vi "main.vi"() -> ()   [LabVIEW 2020]
uses:
  typedefs/typedef_stage_control.ctl
  typedefs/typedef_stage_position.ctl
panel:
  in  "stop":bool
  in  "Stage position":T1
  in  "Stage Control":T2={"Up"=FALSE, "Left"=FALSE, "Right"=FALSE, "Down"=FALSE, "Focus Down"=FALSE, "Focus Up"=FALSE, "X Step Size(um)"=100.0, "Z step size (um)"=100.0, "Y Step Size(um)"=100.0, "Enable x-axis"=TRUE, "Enable y-axis"=TRUE, "Enable z-axis"=TRUE, "Same step size"=FALSE, "Global step size"=0.0, "stop"=FALSE}
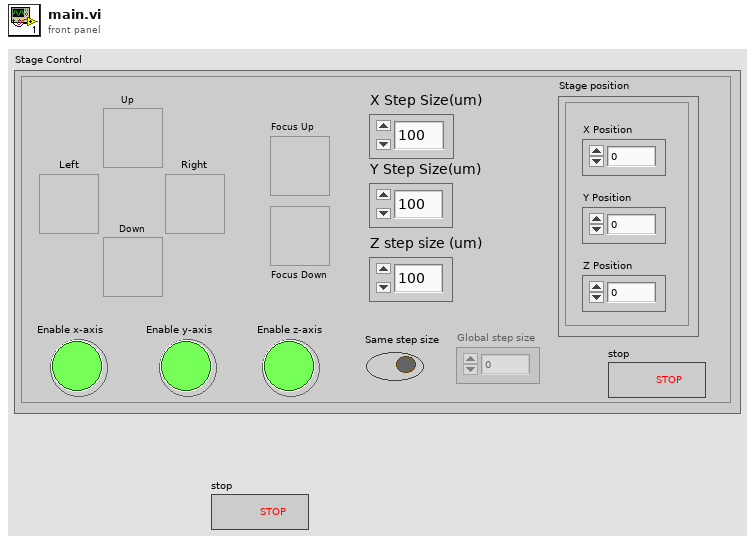
[diagram p1: front panel]
types:
  T1 = typedef "typedef_stage_position.ctl" = cluster{"X Position":dbl, "Y Position":dbl, "Z Position":dbl}
  T2 = typedef "typedef_stage_control.ctl" = cluster{"Up":bool, "Left":bool, "Right":bool, "Down":bool, "Focus Down":bool, "Focus Up":bool, "X Step Size(um)":dbl, "Z step size (um)":dbl, "Y Step Size(um)":dbl, "Enable x-axis":bool, "Enable y-axis":bool, "Enable z-axis":bool, "Same step size":bool, "Global step size":dbl, "stop":bool}
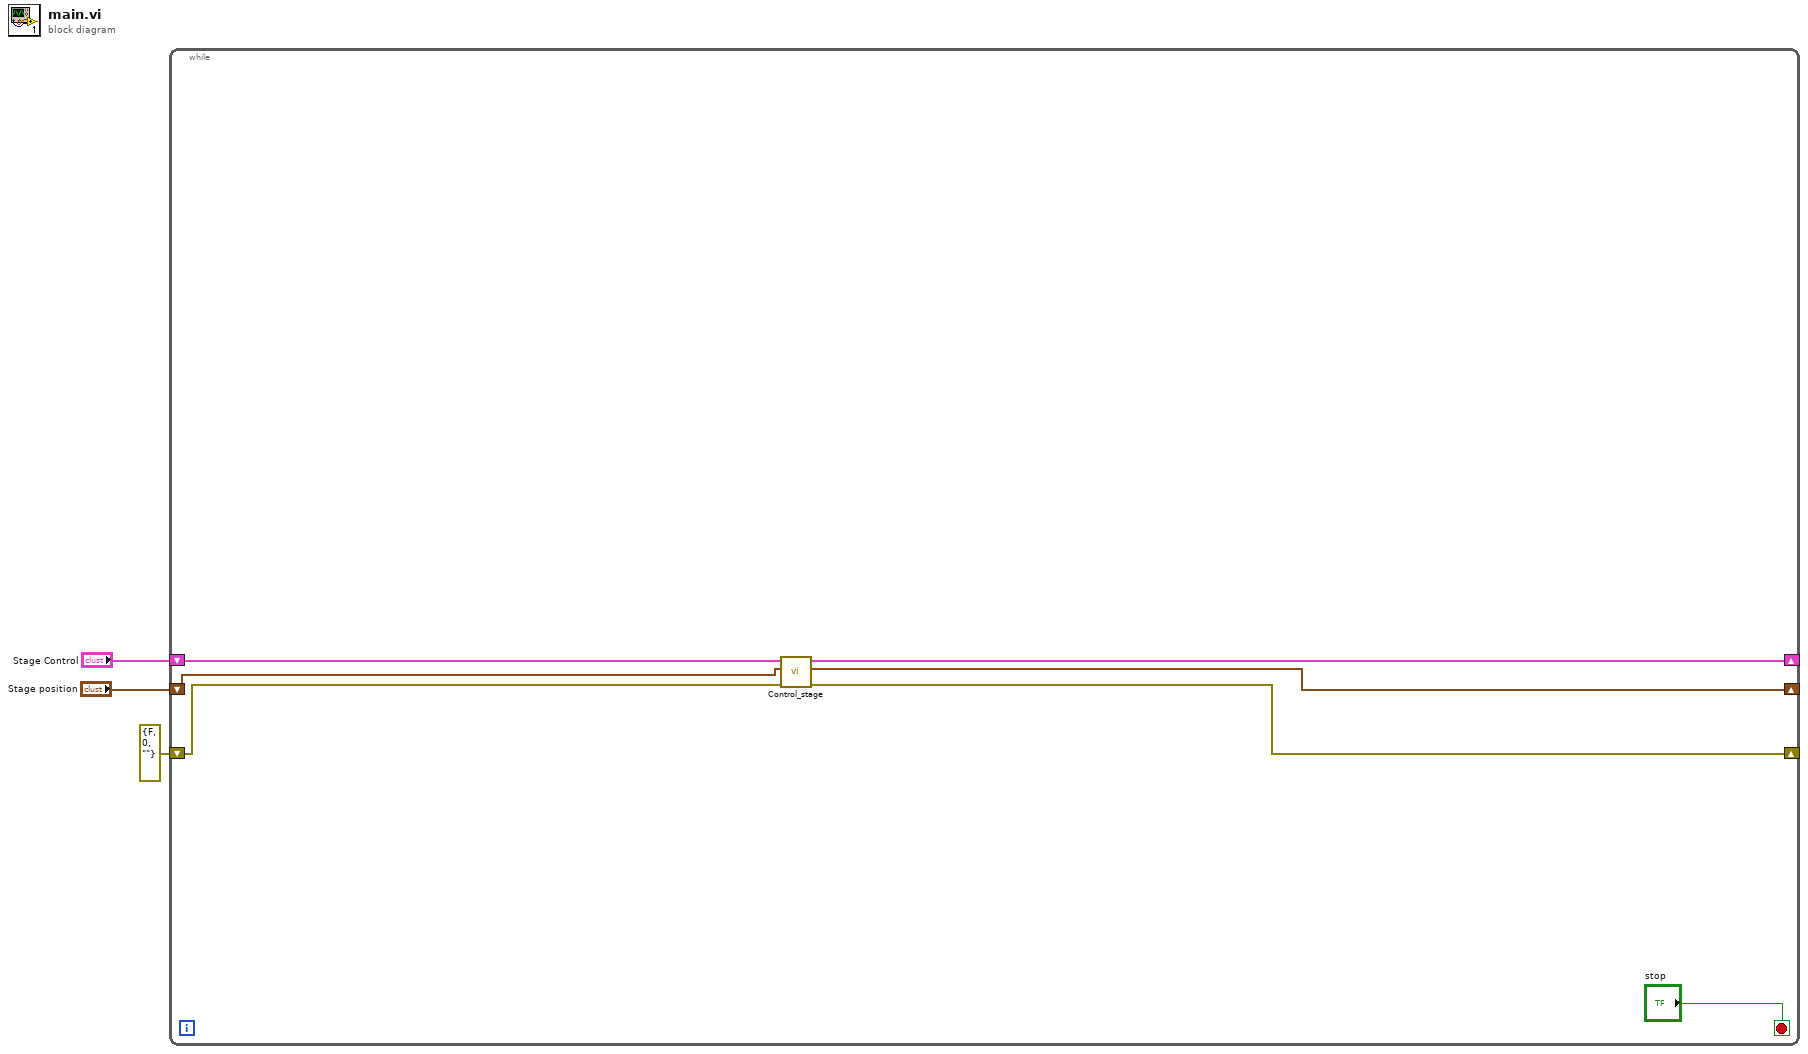
[diagram p0: block diagram]
diagram:
  n1 = while {
    shift-right: [w8] -> _
    shift-left: "Stage Control" -> [w10]
    shift-right: [w7] -> _
    shift-left: "Stage position" -> [w9]
    shift-right: [w6] -> _
    shift-left: errorcluster {"status"=FALSE, "code"=0, "source"=""} ("error out") -> [w5]
    stop <- "stop" stop-if-true
    n2 = call "Control_stage.vi"("error in"=w5, "Stage position IN"=w9, "Stage control IN"=w10) -> ("error out"=w6:errorcluster, "Stage position OUT"=w7:T1, "Stage control OUT"=w8:T2)  [unwired: 6 in]
  }
